vi "CPU_monitoring_test.vi"() -> ()   [LabVIEW 2018]
uses:
  Tracker.lvlib
panel:
  in  "Buffer length, sec":dbl=5.0 min=0.1 max=120.0 step=0.1
  in  "Scan interval, ms":u32=250 min=25 max=5000 step=25
  in  "error in (no error)":errorcluster
  in  "Stop":bool
  out "Waveform Chart":cluster{"CPU load, %":sgl, "mean":dbl}(graph)
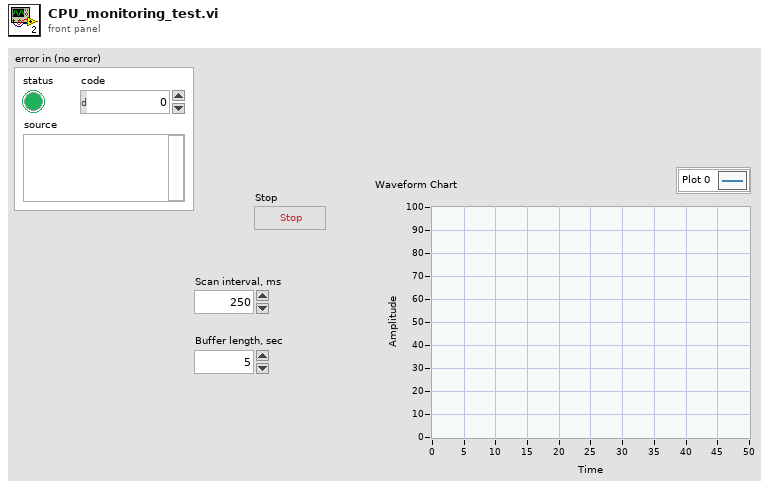
[diagram p1: front panel]
types:
  T1 = cluster{"Instant CPU load, %":sgl, "Historical CPU load, %":sgl}
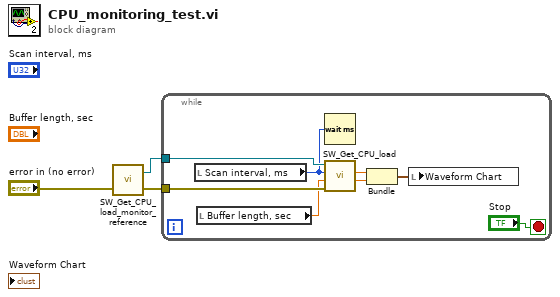
[diagram p0: block diagram]
diagram:
  n1 = call "SW_Get_CPU_load_monitor_reference.vi"("error in (no error)"="error in (no error)") -> ("error out"=w3:errorcluster, "CPU monitor .NET reference"=w2:refnum<k24>)  [unwired: 1 in]
  n2 = while {
    tunnel: w3 -> [w11]
    tunnel: w2 -> [w10]
    stop <- "Stop" stop-if-true
    n3 = local read "Scan interval, ms"() -> (w5:u32)
    n4 = local read "Buffer length, sec"() -> (w4:dbl)
    n5 = Wait (ms)(milliseconds to wait=w5) -> ()  [unwired: 1 out]
    n6 = call "SW_Get_CPU_load.vi"("error in (no error)"=w11, "Buffer length, sec"=w4, "Scan interval, ms"=w5, "CPU monitor .NET reference in"=w10) -> ("Historical CPU load, %"=w7:sgl, "Instant CPU load, %"=w6:sgl)  [unwired: 2 out]
    n7 = Bundle("Instant CPU load, %"=w6, "Historical CPU load, %"=w7) -> (w8:T1)  [unwired: 1 in]
    n8 = local write "Waveform Chart"(w8) -> ()
  }
